vi "speed.vi"() -> ()   [LabVIEW 2020]
uses:
  <vilib>/Quanser/Rapid Control Prototyping Toolkit/hardware/HIL Board/_TypeSpecific/HIL Read Encoder (Scalar).vi
  <vilib>/Quanser/Rapid Control Prototyping Toolkit/hardware/HIL Board/HIL Read Mixed.vi
  <vilib>/Quanser/Rapid Control Prototyping Toolkit/hardware/HIL Board/HIL Close.vi
  <vilib>/Quanser/Rapid Control Prototyping Toolkit/hardware/HIL Board/HIL Board.lvclass
panel:
  out "x/y":dbl
  in  "stop":bool
  out "Waveform Chart":cluster{dbl, dbl}(graph)
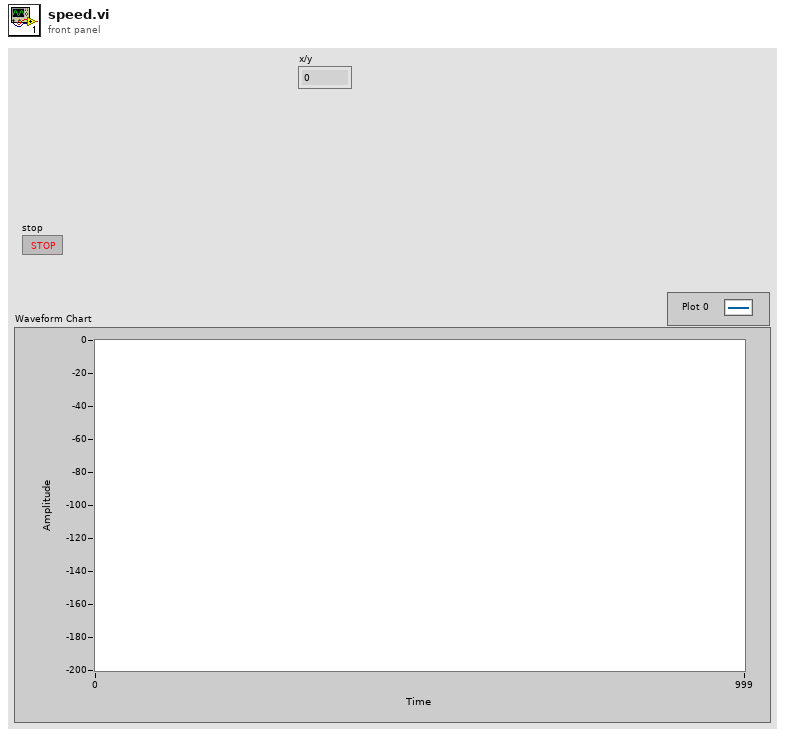
[diagram p1: front panel]
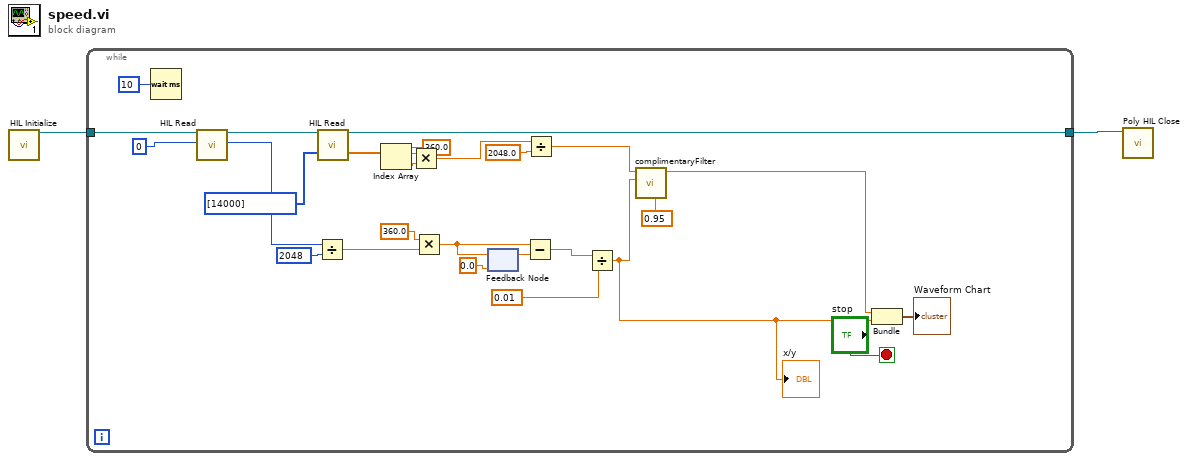
[diagram p0: block diagram]
diagram:
  n1 = call "HIL Initialize"() -> ("board out"=w2:refnum<class "HIL Board.lvclass">)  [unwired: 14 in, 1 out]
  n2 = while {
    tunnel: w2 -> [w18]
    tunnel: [w27] -> w1
    stop <- "stop" stop-if-true
    n3 = Wait (ms)(milliseconds to wait=u32 10) -> ()  [unwired: 1 out]
    n4 = call-poly <vilib>:"HIL Read.vi"("board in"=w18, "channel"=u32 0) -> ("board out"=w7:refnum<class "HIL Board.lvclass">, "counts"=w11:i32)  [unwired: 15 in, 1 out]
    n5 = Divide(x=w11, y=2048) -> (x/y=w16:dbl)
    n6 = call-poly <vilib>:"HIL Read.vi"("board in"=w7, "other channels"=u32[] [14000]) -> ("board out"=w27:refnum<class "HIL Board.lvclass">, "other values"=w25:dbl[])  [unwired: 12 in, 4 out]
    n7 = Index Array(array=w25) -> (element=w21:dbl)  [unwired: 1 in]
    n8 = Multiply(x=360.0, y=w21) -> (x*y=w23:dbl)
    n9 = Multiply(x=360.0, y=w16) -> (x*y=w13:dbl)
    n10 = feedback #1(0.0) -> (w12:dbl)
    n11 = feedback-in #1(w13) -> ()
    n12 = Subtract(x=w13, y=w12) -> (x-y=w10:dbl)
    n13 = Divide(x=w23, y=2048.0) -> (x/y=w6:dbl)
    n14 = Divide(x=w10, y=0.01) -> (x/y=w4:dbl)
    "x/y" <- w4
    n15 = call "complimentaryFilter.vi"("alpha"=0.95, "low pass component"=w4, "high pass component"=w6) -> ("filtered signal"=w5:dbl)  [unwired: 8 in]
    n16 = Bundle("filtered signal"=w5, w4) -> (→"Waveform Chart":cluster{"filtered signal":dbl, dbl})  [unwired: 1 in]
  }
  n17 = call-poly <vilib>:"Poly HIL Close.vi"("board in"=w1) -> ()  [unwired: 10 in, 1 out]
